vi "MemFromHTML_+CreatedTempPath_xPDF.vi"(6 "Identifying_String":string="img src=\"", 8 "error in (no error)":errorcluster, 9 "Dencrypted text":string, 10 "FolderName":string, 11 "Folder_Mgmt":refnum<class "Folder_Mgmt.lvclass">) -> (0 "error out":errorcluster, 1 "ModifyedHTML":string, 2 "TemporaryFiles":path[](array[path]), 3 "Folder_Mgmt 2":refnum<class "Folder_Mgmt.lvclass">)   [LabVIEW 2016, in "Folder_Mgmt.lvclass"]
uses:
  Folder_Mgmt.lvclass
  Folder_Mgmt.lvclass/Folder_Mgmt.ctl
panel:
  out "before substring":string
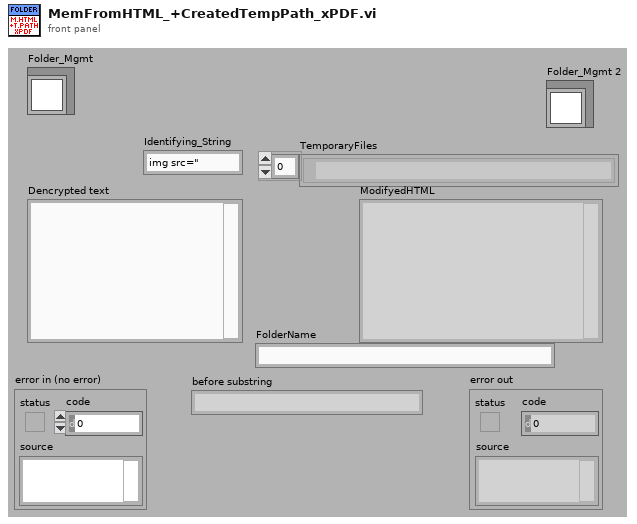
[diagram p1: front panel]
types:
  T1 = enum16{"open", "replace", "create", "open or create", "replace or create", "replace or create with confirmation"}
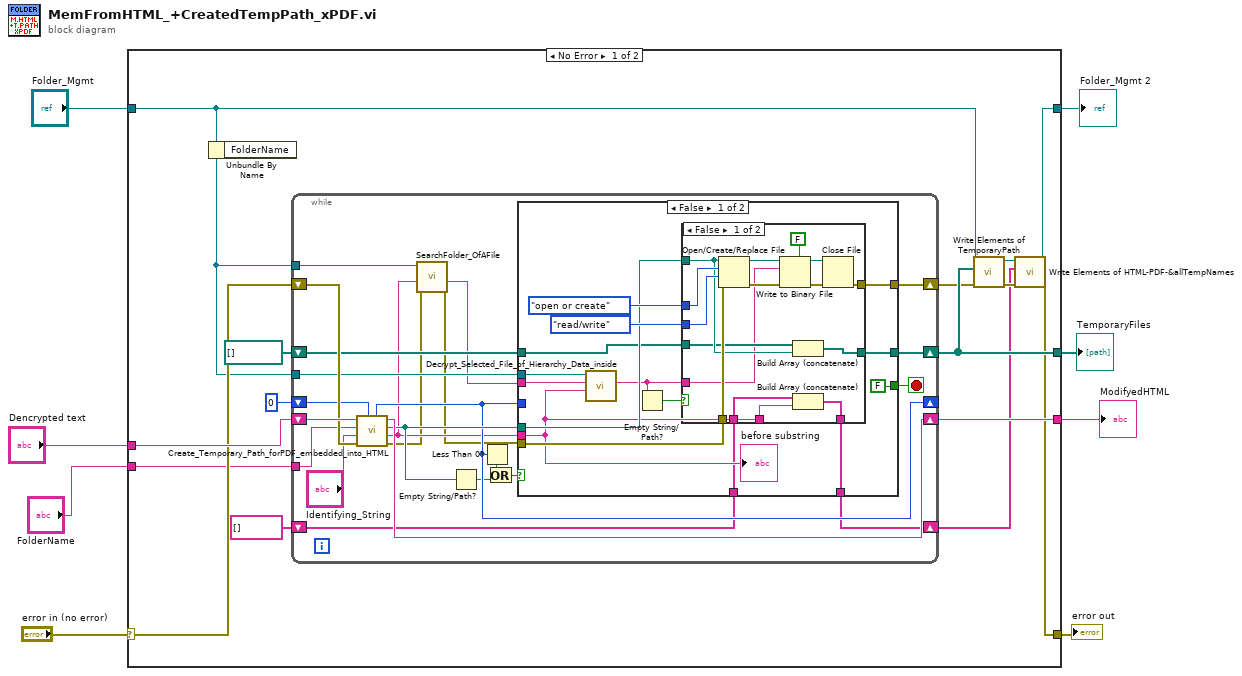
[diagram p0: block diagram]
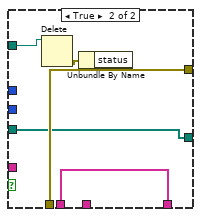
[diagram p2: hidden frame]
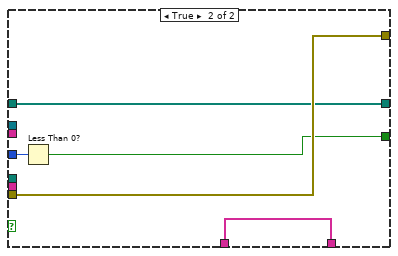
[diagram p3: hidden frame]
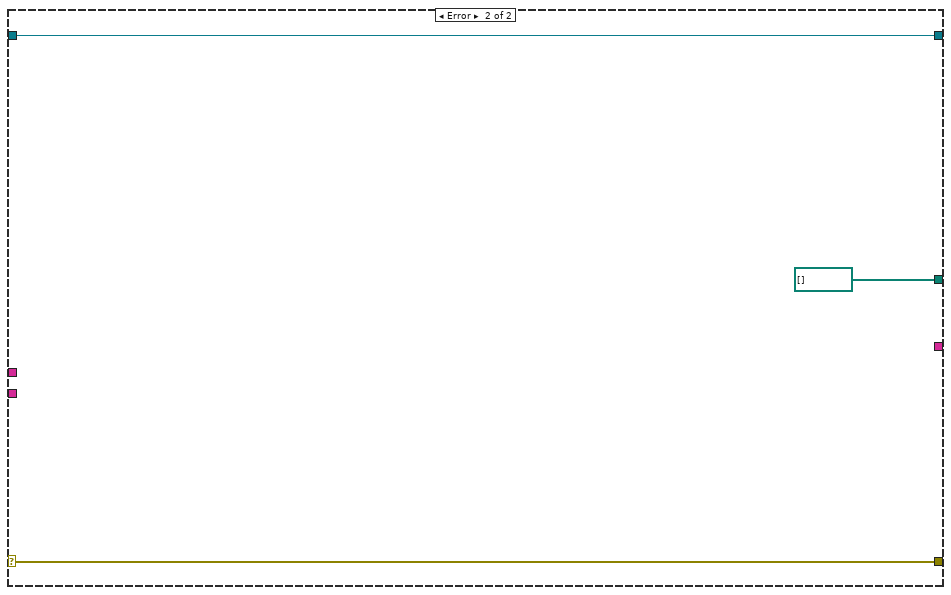
[diagram p4: hidden frame]
diagram:
  n1 = case shown="No Error" "error in (no error)" {
    selector: "error in (no error)" -> [w21 w90]
    tunnel: [w13 w90] -> w7
    tunnel: [w11 w89] -> w3
    tunnel: "Folder_Mgmt" -> [w10 w89]
    tunnel: "Dencrypted text" -> [w22 _]
    tunnel: [w18 path[] []] -> w5
    tunnel: [w20 _] -> w4
    tunnel: "FolderName" -> [w9 _]
    frame No Error {
      n2 = Unbundle By Name(w10) -> ()  [unwired: 1 out]
      n3 = while {
        tunnel: w10 -> [w42]
        shift-right: [w46] -> w17
        shift-left: w21 -> [w43]
        shift-right: [w44] -> w20
        shift-left: w22 -> [w45]
        shift-right: [w36] -> _
        shift-left: 0 ("offset past match") -> [w38]
        shift-right: [w40] -> w18
        shift-left: path[] [] -> [w33]
        shift-right: [w30] -> w14
        shift-left: string[] [] -> [w31]
        tunnel: w10 -> [w29]
        tunnel: w9 -> [w24]
        stop <- w39 stop-if-true
        n4 = call "Create_Temporary_Path_forPDF_embedded_into_HTML.vi"("offset past match"=w38, "error in (no error)"=w43, "Identifying_String"="Identifying_String", "FolderName"=w24, "Dencrypted text"=w45) -> ("error out"=w27:errorcluster, "PDF_fileName"=w28:string, "Temp_PATH"=w41:path, "HTML_wPathChanged"=w44:string, "offset past match"=w36:i32)  [unwired: 2 in]
        n5 = call "SearchFolder_OfAFile.vi"("Folder_Mgmt out"=w29, "FileToSearch"=w28, "error in (no error)"=w27) -> ("FolderOfFile"=w25:string, "error out"=w26:errorcluster)  [unwired: 5 in, 1 out]
        n6 = Empty String/Path?(string/path=w41) -> (empty?=w32:bool)
        n7 = Less Than 0?(x=w36) -> (x < 0?=w35:bool)
        n8 = Or(x=w35, y=w32) -> (x .or. y?=w37:bool)
        n9 = case shown="False" w37 {
          tunnel: [w59 w87] -> w46
          tunnel: w28 -> [w49 _]
          tunnel: w26 -> [w58 w87]
          tunnel: w42 -> [w57 _]
          tunnel: w25 -> [w56 _]
          tunnel: w41 -> [w55 _]
          tunnel: [w53 w86] -> w40
          tunnel: [FALSE w83] -> w39
          tunnel: w36 -> [_ w84]
          tunnel: w33 -> [w52 w86]
          tunnel: w31 -> [w48 w85]
          tunnel: [w47 w85] -> w30
          frame False {
            n10 = call-dynamic "Decrypt_Selected_File_of_Hierarchy_Data_inside.vi"("FileName"=w49, "SubFolderName"=w56, "object in"=w57) -> ("Dencrypted text"=w51:string)  [unwired: 5 in, 3 out]
            n11 = Empty String/Path?(string/path=w51) -> (empty?=w50:bool)
            n12 = case shown="False" w50 {
              tunnel: enum16{"read/write", "read-only", "write-only"}."read/write" ("access (0:read/write)") -> [w73 _]
              tunnel: T1."open or create" ("operation (0:open)") -> [w72 _]
              tunnel: [w70 w82] -> w59
              tunnel: w58 -> [w69 w82]
              tunnel: w55 -> [w68 w80]
              tunnel: [w67 w81] -> w53
              tunnel: w52 -> [w66 w81]
              tunnel: w51 -> [w65 _]
              tunnel: w49 -> [w64 _]
              tunnel: w48 -> [w63 w78]
              tunnel: [w62 w78] -> w47
              frame False {
                n13 = Open/Create/Replace File(file path (use dialog)=w68, error in=w69, operation (0:open)=w72, access (0:read/write)=w73) -> (refnum out=w74:refnum<file>, error out=w75:errorcluster)  [unwired: 2 in, 1 out]
                n14 = Write to Binary File(file (use dialog)=w74, data=w65, error in=w75, 5:FALSE ("prepend array or string size? (T)")) -> (refnum out=w77:refnum<file>, error out=w76:errorcluster)  [unwired: 2 in, 1 out]
                n15 = Build Array (concatenate)(w66, w68) -> (w67:path[])
                n16 = Build Array (concatenate)(w63, w64) -> (w62:string[])
                n17 = Close File(refnum=w77, error in=w76) -> (error out=w70:errorcluster)  [unwired: 1 out]
              }
              frame True {
                n18 = Delete(path (use dialog)=w80) -> (error out=w79:errorcluster)  [unwired: 4 in, 2 out]
                n19 = Unbundle By Name(w79) -> ()  [unwired: 1 out]
              }
            }
            "before substring" <- w49
          }
          frame True {
            n20 = Less Than 0?(x=w84) -> (x < 0?=w83:bool)
          }
        }
      }
      n21 = call "Write Elements of TemporaryPath.vi"("error in (no error)"=w17, "Paths"=w18, "Folder_Mgmt"=w10) -> ("error out"=w15:errorcluster, "Folder_Mgmt 2"=w12:refnum<class "Folder_Mgmt.lvclass">)  [unwired: 7 in]
      n22 = call "Write Elements of HTML-PDF-&allTempNames.vi"("error in (no error)"=w15, "Array"=w14, "Folder_Mgmt"=w12) -> ("error out"=w13:errorcluster, "Folder_Mgmt 2"=w11:refnum<class "Folder_Mgmt.lvclass">)  [unwired: 7 in]
    }
    frame Error {
    }
  }
  "error out" <- w7
  "TemporaryFiles" <- w5
  "ModifyedHTML" <- w4
  "Folder_Mgmt 2" <- w3
